vi "update2D.vi"(8 "error in (no error)":errorcluster, 10 "reshapeInfo":T1, 11 "Image in":T4) -> (0 "error out":errorcluster, 3 "Image out":T4(plugin-control), 5 "time 2Dimage":u32)   [LabVIEW 2013, in "MagAnalysis_Online.lvclass"]
uses:
  MagAnalysis_Online.lvclass
  <vilib>/vision/Image Controls.llb/IMAQ Image.ctl
  reshapeINfo_TypDef.ctl
  emptyArray_TYpDEf.ctl
  emptyArrayCamX_TypDef.ctl
  shared/CompressAndUpdate(Poly)/CompressAndUpdate(Numeric).vi
  shared/CompressAndUpdate(Poly)/CompressAndUpdate(IMAQ Image).vi
  <vilib>/vision/NI_Vision_Development_Module.lvlib
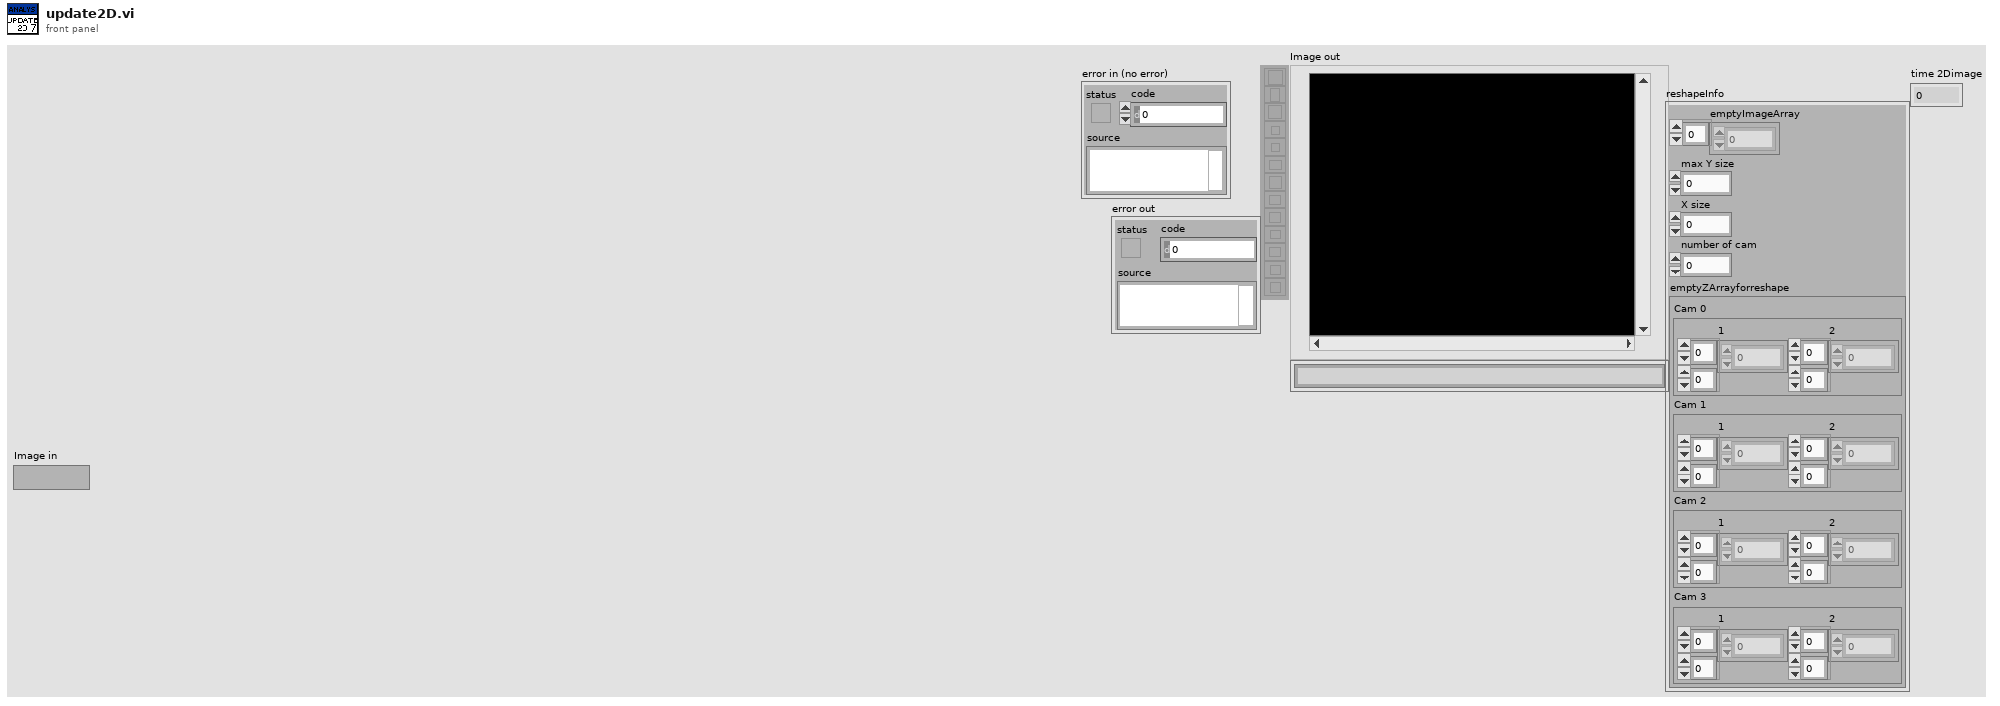
[diagram p1: front panel]
types:
  T1 = typedef "reshapeINfo_TypDef.ctl" = cluster{"emptyImageArray":dbl[], "max Y size":i32, "X size":i32, "number of cam":i32, "emptyZArrayforreshape":T2}
  T2 = typedef "emptyArray_TYpDEf.ctl" = cluster{"Cam 0":T3, "Cam 1":T3, "Cam 2":T3, "Cam 3":T3}
  T3 = typedef "emptyArrayCamX_TypDef.ctl" = cluster{"1":dbl[][], "2":dbl[][]}
  T4 = typedef "IMAQ Image.ctl" = refnum<image>
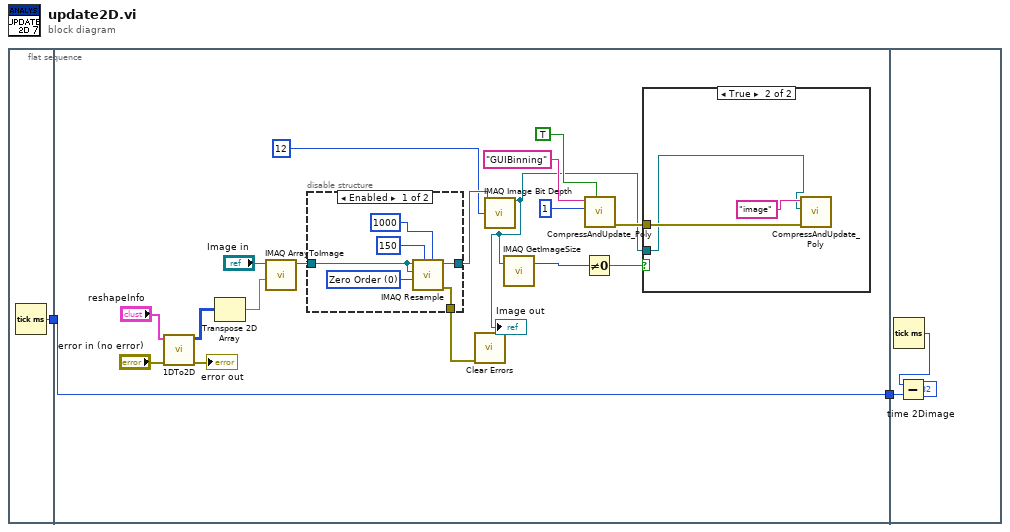
[diagram p0: block diagram]
diagram:
  n1 = flat-sequence {
    tunnel: [w3] -> w1
    tunnel: [w10] -> w2
    tunnel: w1 -> [w10]
    tunnel: w2 -> [w34]
    frame #0 {
      n2 = Tick Count (ms)() -> (millisecond timer value=w3:u32)
    }
    frame #1 {
      n3 = call "1DTo2D.vi"("error in (no error)"="error in (no error)", "reshapeInfo"="reshapeInfo") -> ("error in (no error) 2"=→"error out":errorcluster, "Array out"=w8:i16[][])  [unwired: 8 in]
      n4 = Transpose 2D Array(2D array=w8) -> (transposed array=w7:i16[][])
      n5 = call "IMAQ ArrayToImage"("Image Pixels (I16)"=w7, "Image"="Image in") -> ("Image Out"=w15:T4)  [unwired: 8 in, 1 out]
      n6 = disable-structure shown="Enabled" {
        disable-tunnel: w15 -> [w24 w28]
        disable-tunnel: [w23 w28] -> w6
        disable-tunnel: [w22 _] -> w9
        frame Enabled {
          w25 = u32 0 items=["Zero Order", "Bi-Linear", "Quadratic", "Cubic Spline"] ("Interpolation Type")
          n7 = call "IMAQ Resample"("X Resolution"=1000, "Y Resolution"=150, "Interpolation Type"=w25, "Image Dst"=w24, "Image Src"=w24) -> ("error out"=w22:errorcluster, "Image Dst Out"=w23:T4)  [unwired: 5 in]
        }
        frame Disabled {
        }
      }
      n8 = call <vilib>:"Clear Errors.vi"("error in (no error)"=w9) -> ()  [unwired: 6 in, 1 out]
      n9 = call "IMAQ Image Bit Depth"("Image"=w6, "Bit Depth (0)"=u32 12) -> ("Image Out"=w5:T4)  [unwired: 11 in, 2 out]
      "Image out" <- w5
      n10 = call "IMAQ GetImageSize"("Image"=w5) -> ("Y Resolution"=w19:i32)  [unwired: 3 in, 2 out]
      n11 = Not Equal To 0?(x=w19) -> (x != 0?=w20:bool)
      n12 = call-poly "CompressAndUpdate_Poly.vi"("force CVT update (false)"=TRUE, "Numeric"=1, "command or variable name"="GUIBinning") -> ("error out"=w17:errorcluster)  [unwired: 8 in]
      n13 = case shown="True" w20 {
        tunnel: w17 -> [_ w31]
        tunnel: w5 -> [_ w29]
        frame False {
        }
        frame True {
          n14 = call-poly "CompressAndUpdate_Poly.vi"("error in"=w31, "IMAQ Image"=w29, "command or variable name"="image") -> ()  [unwired: 8 in, 1 out]
        }
      }
    }
    frame #2 {
      n15 = Tick Count (ms)() -> (millisecond timer value=w33:u32)
      n16 = Subtract(x=w33, y=w34) -> (x-y=→"time 2Dimage":u32)
    }
  }
